vi "module template new.vi"(0 "Static input":T4(array[cluster])=[{"Times"=[947.0, 994.5, 1000.0], "Voltages"=[2.0, -0.5, 2.0], "Enable Ch"=TRUE, "Hinge Points"=3}, {"Times"=[947.0, 994.5, 1000.0], "Voltages"=[-1.0, 0.0, 2.0], "Enable Ch"=TRUE, "Hinge Points"=3}, {"Times"=[947.0, 994.5, 1000.0], "Voltages"=[2.0, -1.0, 2.0], "Enable Ch"=TRUE, "Hinge Points"=3}, {"Times"=[948.5, 1000.0], "Voltages"=[0.05, 0.0], "Enable Ch"=TRUE, "Hinge Points"=2}, {"Times"=[1000.0, 2850.0], "Voltages"=[8.0, -0.5], "Enable Ch"=TRUE, "Hinge Points"=2}, {"Times"=[947.0, 1000.0], "Voltages"=[4.6, 4.3], "Enable Ch"=TRUE, "Hinge Points"=2}, {"Times"=[996.0, 999.0, 1400.0, 1402.0, 1404.0, 1406.0, 1408.0, 1410.0, 1412.0, 1414.0, 1416.0, 1418.0, 1420.0, 1422.0, 1424.0, 1426.0, 1428.0, 1430.0, 1432.0, 1434.0, 1436.0, 1438.0, 1440.0, 1442.0, 1444.0, 1446.0, 1448.0, 1450.0, 1452.0, 1454.0, 1456.0, 1458.0, 1460.0, 1462.0, 1464.0, 1466.0, 1468.0, 1470.0, 1472.0, 1474.0, 1476.0, 1478.0, 1480.0, 1482.0, 1484.0, 1486.0, 1488.0, 1490.0, 1492.0, 1494.0, 1496.0, 1498.0, 1500.0], "Voltages"=[0.0, -1.2, -1.2, -1.256, -1.3119999999999998, -1.3679999999999999, -1.424, -1.48, -1.536, -1.5919999999999999, -1.648, -1.704, -1.7599999999999998, -1.8159999999999998, -1.8719999999999999, -1.928, -1.984, -2.04, -2.096, -2.152, -2.208, -2.264, -2.32, -2.376, -2.4319999999999995, -2.4879999999999995, -2.5439999999999996, -2.5999999999999996, -2.6559999999999997, -2.7119999999999997, -2.768, -2.824, -2.88, -2.936, -2.992, -3.048, -3.104, -3.1599999999999997, -3.216, -3.2719999999999994, -3.3279999999999994, -3.3839999999999995, -3.4399999999999995, -3.4959999999999996, -3.5519999999999996, -3.6079999999999997, -3.6639999999999997, -3.7199999999999998, -3.776, -3.832, -3.888, -3.944, -4.0], "Enable Ch"=TRUE, "Hinge Points"=53}, {"Times"=[], "Voltages"=[], "Enable Ch"=FALSE, "Hinge Points"=0}, {"Times"=[], "Voltages"=[], "Enable Ch"=FALSE, "Hinge Points"=0}, {"Times"=[], "Voltages"=[], "Enable Ch"=FALSE, "Hinge Points"=0}, {"Times"=[], "Voltages"=[], "Enable Ch"=FALSE, "Hinge Points"=0}, {"Times"=[], "Voltages"=[], "Enable Ch"=FALSE, "Hinge Points"=0}, {"Times"=[], "Voltages"=[], "Enable Ch"=FALSE, "Hinge Points"=0}, {"Times"=[], "Voltages"=[], "Enable Ch"=FALSE, "Hinge Points"=0}, {"Times"=[], "Voltages"=[], "Enable Ch"=FALSE, "Hinge Points"=0}, {"Times"=[], "Voltages"=[], "Enable Ch"=FALSE, "Hinge Points"=0}] {"Voltages" format="%.2f"; "Times" format="%.2f"}, 1 "Absolute start time (ms)":dbl=2900.0 format="%.3f", 2 "GPIB Input":T1(array[cluster]) {"Module" items=["TTL high                                                                                 ", "TTL low                          ", "Camera Strobe                   ", "CMOT", "Defaults                           ", "Fluorescence pulse           ", "IP trap                         ", "Kinetics OD image          ", "Kinetics picture", "Kinetics probe pulse", "MOT light only                ", "MOT off                                   ", "MOT on                         ", "Move cart                      ", "OD image                     ", "Optical pumping          ", "Picture                             ", "Probe Pulse", "Quadrupole trap             ", "IP off", "Utility Module 02           ", "Utility Module 03           ", "Molasses          ", "Utility Module 04     ", "Utility Module 05     ", "Utility Module 06     ", "Utility Module 07     ", "Utility Module 08     ", "Utility Module 09     ", "Utility Module 10     ", "Static DAC", "GPIB"]; "Abs Start Time" format="%.3f"}, 3 "Read/Write":bool, 5 "Input":i32[][](array[numeric])=[[-1000, 0, 15, 0], [100, 3, 14, 1], [10000, 3, 14, 0], [947000, 0, 11, 1], [947000, 1, 13, 0], [947000, 2, 9, 1], [947000, 2, 9, 1], [947000, 2, 9, 1], [947000, 2, 9, 1], [947100, 2, 9, 0], [947100, 2, 9, 0], [947100, 2, 9, 0], [947100, 2, 9, 0], [948500, 2, 9, 1], [948600, 2, 9, 0], [990000, 0, 0, 0], [992000, 2, 11, 0], [992000, 2, 12, 1], [994000, 0, 9, 0], [994000, 2, 2, 0], [994500, 2, 9, 1], [994500, 2, 9, 1], [994500, 2, 9, 1], [994600, 2, 9, 0], [994600, 2, 9, 0], [994600, 2, 9, 0], [995500, 1, 0, 0], [996000, 2, 9, 1], [996100, 2, 9, 0], [996500, 0, 5, 0], [996500, 1, 1, 0], [996500, 1, 9, 0], [996500, 2, 3, 1], [997000, 0, 3, 1], [998300, 0, 3, 0], [998450, 0, 11, 0], [998450, 1, 13, 1], [998500, 0, 4, 1], [998850, 0, 14, 1], [999000, 2, 9, 1], [999100, 2, 9, 0], [999450, 0, 14, 0], [999500, 0, 4, 0], [999500, 0, 15, 1], [1000000, 0, 0, 1], [1000000, 0, 1, 1], [1000000, 0, 2, 1], [1000000, 0, 5, 1], [1000000, 1, 1, 1], [1000000, 1, 9, 1], [1000000, 2, 7, 1], [1000000, 2, 9, 1], [1000000, 2, 9, 1], [1000000, 2, 9, 1], [1000000, 2, 9, 1], [1000000, 2, 9, 1], [1000000, 2, 9, 1], [1000100, 2, 9, 0], [1000100, 2, 9, 0], [1000100, 2, 9, 0], [1000100, 2, 9, 0], [1000100, 2, 9, 0], [1000100, 2, 9, 0], [1000500, 2, 3, 0], [1001000, 2, 7, 0], [1005000, 0, 2, 0], [1047000, 2, 11, 0], [1047000, 2, 12, 0], [1400000, 2, 9, 1], [1400100, 2, 9, 0], [1402000, 2, 9, 1], [1402100, 2, 9, 0], [1404000, 2, 9, 1], [1404100, 2, 9, 0], [1406000, 2, 9, 1], [1406100, 2, 9, 0], [1408000, 2, 9, 1], [1408100, 2, 9, 0], [1410000, 2, 9, 1], [1410100, 2, 9, 0], [1412000, 2, 9, 1], [1412100, 2, 9, 0], [1414000, 2, 9, 1], [1414100, 2, 9, 0], [1416000, 2, 9, 1], [1416100, 2, 9, 0], [1418000, 2, 9, 1], [1418100, 2, 9, 0], [1420000, 2, 9, 1], [1420100, 2, 9, 0], [1422000, 2, 9, 1], [1422100, 2, 9, 0], [1424000, 2, 9, 1], [1424100, 2, 9, 0], [1426000, 2, 9, 1], [1426100, 2, 9, 0], [1428000, 2, 9, 1], [1428100, 2, 9, 0], [1430000, 2, 9, 1], [1430100, 2, 9, 0], [1432000, 2, 9, 1], [1432100, 2, 9, 0], [1434000, 2, 9, 1], [1434100, 2, 9, 0], [1436000, 2, 9, 1], [1436100, 2, 9, 0], [1438000, 2, 9, 1], [1438100, 2, 9, 0], [1440000, 2, 9, 1], [1440100, 2, 9, 0], [1442000, 2, 9, 1], [1442100, 2, 9, 0], [1444000, 2, 9, 1], [1444100, 2, 9, 0], [1446000, 2, 9, 1], [1446100, 2, 9, 0], [1448000, 2, 9, 1], [1448100, 2, 9, 0], [1450000, 2, 9, 1], [1450100, 2, 9, 0], [1452000, 2, 9, 1], [1452100, 2, 9, 0], [1454000, 2, 9, 1], [1454100, 2, 9, 0], [1456000, 2, 9, 1], [1456100, 2, 9, 0], [1458000, 2, 9, 1], [1458100, 2, 9, 0], [1460000, 2, 9, 1], [1460100, 2, 9, 0], [1462000, 2, 9, 1], [1462100, 2, 9, 0], [1464000, 2, 9, 1], [1464100, 2, 9, 0], [1466000, 2, 9, 1], [1466100, 2, 9, 0], [1468000, 2, 9, 1], [1468100, 2, 9, 0], [1470000, 2, 9, 1], [1470100, 2, 9, 0], [1472000, 2, 9, 1], [1472100, 2, 9, 0], [1474000, 2, 9, 1], [1474100, 2, 9, 0], [1476000, 2, 9, 1], [1476100, 2, 9, 0], [1478000, 2, 9, 1], [1478100, 2, 9, 0], [1480000, 2, 9, 1], [1480100, 2, 9, 0], [1482000, 2, 9, 1], [1482100, 2, 9, 0], [1484000, 2, 9, 1], [1484100, 2, 9, 0], [1486000, 2, 9, 1], [1486100, 2, 9, 0], [1488000, 2, 9, 1], [1488100, 2, 9, 0], [1490000, 2, 9, 1], [1490100, 2, 9, 0], [1492000, 2, 9, 1], [1492100, 2, 9, 0], [1494000, 2, 9, 1], [1494100, 2, 9, 0], [1496000, 2, 9, 1], [1496100, 2, 9, 0], [1498000, 2, 9, 1], [1498100, 2, 9, 0], [1500000, 2, 9, 1], [1500100, 2, 9, 0], [2400000, 0, 1, 0], [2850000, 2, 9, 1], [2850100, 2, 9, 0]], 7 "Static DAC Linear Ramps":T3(array[cluster])=[{"Write Ramp?"=TRUE, "DAC Channel"=6, "Ramp begin"=400.0, "Ramp end"=500.0, "start value"=-1.2, "end value"=-4.0, "steps"=50}] {"end value" format="%_6g"; "start value" format="%_6g"; "Ramp end" format="%_6g"; "Ramp begin" format="%_6g"; "DAC Channel" items=["0", "1", "2", "3", "4", "5", "6", "7", "8", "9", "10", "11", "12", "13", "14", "0"]}, 9 "Manual Array":T5(array[cluster])=[{"Time2 (ms)"=0.0, "Port2"=1, "Line2"=1, "Comments2"="master switch to coils on", "Value2"=TRUE, "Enable2"=TRUE, "DAC value"=0.0}, {"Time2 (ms)"=-1.0, "Port2"=4, "Line2"=6, "Comments2"="Q trap current to 120A", "Value2"=FALSE, "Enable2"=TRUE, "DAC value"=-1.2}, {"Time2 (ms)"=0.0, "Port2"=4, "Line2"=0, "Comments2"="E/W shim off for Qtrap", "Value2"=FALSE, "Enable2"=TRUE, "DAC value"=2.0}, {"Time2 (ms)"=0.0, "Port2"=4, "Line2"=1, "Comments2"="U/D shim off for Qtrap", "Value2"=FALSE, "Enable2"=TRUE, "DAC value"=2.0}, {"Time2 (ms)"=0.0, "Port2"=4, "Line2"=2, "Comments2"="N/S shim off for Qtrap", "Value2"=FALSE, "Enable2"=TRUE, "DAC value"=2.0}, {"Time2 (ms)"=0.0, "Port2"=0, "Line2"=2, "Comments2"="fast turn on (IGBT on)", "Value2"=TRUE, "Enable2"=TRUE, "DAC value"=0.0}, {"Time2 (ms)"=5.0, "Port2"=0, "Line2"=2, "Comments2"="IGBT off", "Value2"=FALSE, "Enable2"=TRUE, "DAC value"=0.0}] {"Line2" items=["0", "1", "2", "3", "4", "5", "6", "7", "8", "9", "10", "11", "12", "13", "14", "15"]; "Port2" items=["A", "B", "C", "D", "DAC", "GPIB"]; "Time2 (ms)" format="%.3f"}, 10 "Do Write/Read":bool, 12 "Do this?":bool=TRUE, 14 "filename":string="quad trap") -> (4 "Static output":T4(array[cluster])=[{"Times"=[947.0, 994.5, 1000.0, 2900.0], "Voltages"=[2.0, -0.5, 2.0, 2.0], "Enable Ch"=TRUE, "Hinge Points"=4}, {"Times"=[947.0, 994.5, 1000.0, 2900.0], "Voltages"=[-1.0, 0.0, 2.0, 2.0], "Enable Ch"=TRUE, "Hinge Points"=4}, {"Times"=[947.0, 994.5, 1000.0, 2900.0], "Voltages"=[2.0, -1.0, 2.0, 2.0], "Enable Ch"=TRUE, "Hinge Points"=4}, {"Times"=[948.5, 1000.0], "Voltages"=[0.05, 0.0], "Enable Ch"=TRUE, "Hinge Points"=2}, {"Times"=[1000.0, 2850.0], "Voltages"=[8.0, -0.5], "Enable Ch"=TRUE, "Hinge Points"=2}, {"Times"=[947.0, 1000.0], "Voltages"=[4.6, 4.3], "Enable Ch"=TRUE, "Hinge Points"=2}, {"Times"=[996.0, 999.0, 1400.0, 1402.0, 1404.0, 1406.0, 1408.0, 1410.0, 1412.0, 1414.0, 1416.0, 1418.0, 1420.0, 1422.0, 1424.0, 1426.0, 1428.0, 1430.0, 1432.0, 1434.0, 1436.0, 1438.0, 1440.0, 1442.0, 1444.0, 1446.0, 1448.0, 1450.0, 1452.0, 1454.0, 1456.0, 1458.0, 1460.0, 1462.0, 1464.0, 1466.0, 1468.0, 1470.0, 1472.0, 1474.0, 1476.0, 1478.0, 1480.0, 1482.0, 1484.0, 1486.0, 1488.0, 1490.0, 1492.0, 1494.0, 1496.0, 1498.0, 1500.0, 2899.0, 3300.0, 3302.0, 3304.0, 3306.0, 3308.0, 3310.0, 3312.0, 3314.0, 3316.0, 3318.0, 3320.0, 3322.0, 3324.0, 3326.0, 3328.0, 3330.0, 3332.0, 3334.0, 3336.0, 3338.0, 3340.0, 3342.0, 3344.0, 3346.0, 3348.0, 3350.0, 3352.0, 3354.0, 3356.0, 3358.0, 3360.0, 3362.0, 3364.0, 3366.0, 3368.0, 3370.0, 3372.0, 3374.0, 3376.0, 3378.0, 3380.0, 3382.0, 3384.0, 3386.0, 3388.0, 3390.0, 3392.0, 3394.0, 3396.0, 3398.0, 3400.0], "Voltages"=[0.0, -1.2, -1.2, -1.256, -1.3119999999999998, -1.3679999999999999, -1.424, -1.48, -1.536, -1.5919999999999999, -1.648, -1.704, -1.7599999999999998, -1.8159999999999998, -1.8719999999999999, -1.928, -1.984, -2.04, -2.096, -2.152, -2.208, -2.264, -2.32, -2.376, -2.4319999999999995, -2.4879999999999995, -2.5439999999999996, -2.5999999999999996, -2.6559999999999997, -2.7119999999999997, -2.768, -2.824, -2.88, -2.936, -2.992, -3.048, -3.104, -3.1599999999999997, -3.216, -3.2719999999999994, -3.3279999999999994, -3.3839999999999995, -3.4399999999999995, -3.4959999999999996, -3.5519999999999996, -3.6079999999999997, -3.6639999999999997, -3.7199999999999998, -3.776, -3.832, -3.888, -3.944, -4.0, -1.2, -1.2, -1.256, -1.3119999999999998, -1.3679999999999999, -1.424, -1.48, -1.536, -1.5919999999999999, -1.648, -1.704, -1.7599999999999998, -1.8159999999999998, -1.8719999999999999, -1.928, -1.984, -2.04, -2.096, -2.152, -2.208, -2.264, -2.32, -2.376, -2.4319999999999995, -2.4879999999999995, -2.5439999999999996, -2.5999999999999996, -2.6559999999999997, -2.7119999999999997, -2.768, -2.824, -2.88, -2.936, -2.992, -3.048, -3.104, -3.1599999999999997, -3.216, -3.2719999999999994, -3.3279999999999994, -3.3839999999999995, -3.4399999999999995, -3.4959999999999996, -3.5519999999999996, -3.6079999999999997, -3.6639999999999997, -3.7199999999999998, -3.776, -3.832, -3.888, -3.944, -4.0], "Enable Ch"=TRUE, "Hinge Points"=105}, {"Times"=[], "Voltages"=[], "Enable Ch"=FALSE, "Hinge Points"=0}, {"Times"=[], "Voltages"=[], "Enable Ch"=FALSE, "Hinge Points"=0}, {"Times"=[], "Voltages"=[], "Enable Ch"=FALSE, "Hinge Points"=0}, {"Times"=[], "Voltages"=[], "Enable Ch"=FALSE, "Hinge Points"=0}, {"Times"=[], "Voltages"=[], "Enable Ch"=FALSE, "Hinge Points"=0}, {"Times"=[], "Voltages"=[], "Enable Ch"=FALSE, "Hinge Points"=0}, {"Times"=[], "Voltages"=[], "Enable Ch"=FALSE, "Hinge Points"=0}, {"Times"=[], "Voltages"=[], "Enable Ch"=FALSE, "Hinge Points"=0}, {"Times"=[], "Voltages"=[], "Enable Ch"=FALSE, "Hinge Points"=0}] {"Voltages" format="%.2f"; "Times" format="%.2f"}, 6 "Output":i32[][](array[numeric])=[[3400100, 2, 9, 0], [3400000, 2, 9, 1], [3398100, 2, 9, 0], [3398000, 2, 9, 1], [3396100, 2, 9, 0], [3396000, 2, 9, 1], [3394100, 2, 9, 0], [3394000, 2, 9, 1], [3392100, 2, 9, 0], [3392000, 2, 9, 1], [3390100, 2, 9, 0], [3390000, 2, 9, 1], [3388100, 2, 9, 0], [3388000, 2, 9, 1], [3386100, 2, 9, 0], [3386000, 2, 9, 1], [3384100, 2, 9, 0], [3384000, 2, 9, 1], [3382100, 2, 9, 0], [3382000, 2, 9, 1], [3380100, 2, 9, 0], [3380000, 2, 9, 1], [3378100, 2, 9, 0], [3378000, 2, 9, 1], [3376100, 2, 9, 0], [3376000, 2, 9, 1], [3374100, 2, 9, 0], [3374000, 2, 9, 1], [3372100, 2, 9, 0], [3372000, 2, 9, 1], [3370100, 2, 9, 0], [3370000, 2, 9, 1], [3368100, 2, 9, 0], [3368000, 2, 9, 1], [3366100, 2, 9, 0], [3366000, 2, 9, 1], [3364100, 2, 9, 0], [3364000, 2, 9, 1], [3362100, 2, 9, 0], [3362000, 2, 9, 1], [3360100, 2, 9, 0], [3360000, 2, 9, 1], [3358100, 2, 9, 0], [3358000, 2, 9, 1], [3356100, 2, 9, 0], [3356000, 2, 9, 1], [3354100, 2, 9, 0], [3354000, 2, 9, 1], [3352100, 2, 9, 0], [3352000, 2, 9, 1], [3350100, 2, 9, 0], [3350000, 2, 9, 1], [3348100, 2, 9, 0], [3348000, 2, 9, 1], [3346100, 2, 9, 0], [3346000, 2, 9, 1], [3344100, 2, 9, 0], [3344000, 2, 9, 1], [3342100, 2, 9, 0], [3342000, 2, 9, 1], [3340100, 2, 9, 0], [3340000, 2, 9, 1], [3338100, 2, 9, 0], [3338000, 2, 9, 1], [3336100, 2, 9, 0], [3336000, 2, 9, 1], [3334100, 2, 9, 0], [3334000, 2, 9, 1], [3332100, 2, 9, 0], [3332000, 2, 9, 1], [3330100, 2, 9, 0], [3330000, 2, 9, 1], [3328100, 2, 9, 0], [3328000, 2, 9, 1], [3326100, 2, 9, 0], [3326000, 2, 9, 1], [3324100, 2, 9, 0], [3324000, 2, 9, 1], [3322100, 2, 9, 0], [3322000, 2, 9, 1], [3320100, 2, 9, 0], [3320000, 2, 9, 1], [3318100, 2, 9, 0], [3318000, 2, 9, 1], [3316100, 2, 9, 0], [3316000, 2, 9, 1], [3314100, 2, 9, 0], [3314000, 2, 9, 1], [3312100, 2, 9, 0], [3312000, 2, 9, 1], [3310100, 2, 9, 0], [3310000, 2, 9, 1], [3308100, 2, 9, 0], [3308000, 2, 9, 1], [3306100, 2, 9, 0], [3306000, 2, 9, 1], [3304100, 2, 9, 0], [3304000, 2, 9, 1], [3302100, 2, 9, 0], [3302000, 2, 9, 1], [3300100, 2, 9, 0], [3300000, 2, 9, 1], [2900100, 2, 9, 0], [2900000, 2, 9, 1], [2900100, 2, 9, 0], [2900000, 2, 9, 1], [2900100, 2, 9, 0], [2900000, 2, 9, 1], [2899100, 2, 9, 0], [2899000, 2, 9, 1], [-1000, 0, 15, 0], [100, 3, 14, 1], [10000, 3, 14, 0], [947000, 0, 11, 1], [947000, 1, 13, 0], [947000, 2, 9, 1], [947000, 2, 9, 1], [947000, 2, 9, 1], [947000, 2, 9, 1], [947100, 2, 9, 0], [947100, 2, 9, 0], [947100, 2, 9, 0], [947100, 2, 9, 0], [948500, 2, 9, 1], [948600, 2, 9, 0], [990000, 0, 0, 0], [992000, 2, 11, 0], [992000, 2, 12, 1], [994000, 0, 9, 0], [994000, 2, 2, 0], [994500, 2, 9, 1], [994500, 2, 9, 1], [994500, 2, 9, 1], [994600, 2, 9, 0], [994600, 2, 9, 0], [994600, 2, 9, 0], [995500, 1, 0, 0], [996000, 2, 9, 1], [996100, 2, 9, 0], [996500, 0, 5, 0], [996500, 1, 1, 0], [996500, 1, 9, 0], [996500, 2, 3, 1], [997000, 0, 3, 1], [998300, 0, 3, 0], [998450, 0, 11, 0], [998450, 1, 13, 1], [998500, 0, 4, 1], [998850, 0, 14, 1], [999000, 2, 9, 1], [999100, 2, 9, 0], [999450, 0, 14, 0], [999500, 0, 4, 0], [999500, 0, 15, 1], [1000000, 0, 0, 1], [1000000, 0, 1, 1], [1000000, 0, 2, 1], [1000000, 0, 5, 1], [1000000, 1, 1, 1], [1000000, 1, 9, 1], [1000000, 2, 7, 1], [1000000, 2, 9, 1], [1000000, 2, 9, 1], [1000000, 2, 9, 1], [1000000, 2, 9, 1], [1000000, 2, 9, 1], [1000000, 2, 9, 1], [1000100, 2, 9, 0], [1000100, 2, 9, 0], [1000100, 2, 9, 0], [1000100, 2, 9, 0], [1000100, 2, 9, 0], [1000100, 2, 9, 0], [1000500, 2, 3, 0], [1001000, 2, 7, 0], [1005000, 0, 2, 0], [1047000, 2, 11, 0], [1047000, 2, 12, 0], [1400000, 2, 9, 1], [1400100, 2, 9, 0], [1402000, 2, 9, 1], [1402100, 2, 9, 0], [1404000, 2, 9, 1], [1404100, 2, 9, 0], [1406000, 2, 9, 1], [1406100, 2, 9, 0], [1408000, 2, 9, 1], [1408100, 2, 9, 0], [1410000, 2, 9, 1], [1410100, 2, 9, 0], [1412000, 2, 9, 1], [1412100, 2, 9, 0], [1414000, 2, 9, 1], [1414100, 2, 9, 0], [1416000, 2, 9, 1], [1416100, 2, 9, 0], [1418000, 2, 9, 1], [1418100, 2, 9, 0], [1420000, 2, 9, 1], [1420100, 2, 9, 0], [1422000, 2, 9, 1], [1422100, 2, 9, 0], [1424000, 2, 9, 1], [1424100, 2, 9, 0], [1426000, 2, 9, 1], [1426100, 2, 9, 0], [1428000, 2, 9, 1], [1428100, 2, 9, 0], [1430000, 2, 9, 1], [1430100, 2, 9, 0], [1432000, 2, 9, 1], [1432100, 2, 9, 0], [1434000, 2, 9, 1], [1434100, 2, 9, 0], [1436000, 2, 9, 1], [1436100, 2, 9, 0], [1438000, 2, 9, 1], [1438100, 2, 9, 0], [1440000, 2, 9, 1], [1440100, 2, 9, 0], [1442000, 2, 9, 1], [1442100, 2, 9, 0], [1444000, 2, 9, 1], [1444100, 2, 9, 0], [1446000, 2, 9, 1], [1446100, 2, 9, 0], [1448000, 2, 9, 1], [1448100, 2, 9, 0], [1450000, 2, 9, 1], [1450100, 2, 9, 0], [1452000, 2, 9, 1], [1452100, 2, 9, 0], [1454000, 2, 9, 1], [1454100, 2, 9, 0], [1456000, 2, 9, 1], [1456100, 2, 9, 0], [1458000, 2, 9, 1], [1458100, 2, 9, 0], [1460000, 2, 9, 1], [1460100, 2, 9, 0], [1462000, 2, 9, 1], [1462100, 2, 9, 0], [1464000, 2, 9, 1], [1464100, 2, 9, 0], [1466000, 2, 9, 1], [1466100, 2, 9, 0], [1468000, 2, 9, 1], [1468100, 2, 9, 0], [1470000, 2, 9, 1], [1470100, 2, 9, 0], [1472000, 2, 9, 1], [1472100, 2, 9, 0], [1474000, 2, 9, 1], [1474100, 2, 9, 0], [1476000, 2, 9, 1], [1476100, 2, 9, 0], [1478000, 2, 9, 1], [1478100, 2, 9, 0], [1480000, 2, 9, 1], [1480100, 2, 9, 0], [1482000, 2, 9, 1], [1482100, 2, 9, 0], [1484000, 2, 9, 1], [1484100, 2, 9, 0], [1486000, 2, 9, 1], [1486100, 2, 9, 0], [1488000, 2, 9, 1], [1488100, 2, 9, 0], [1490000, 2, 9, 1], [1490100, 2, 9, 0], [1492000, 2, 9, 1], [1492100, 2, 9, 0], [1494000, 2, 9, 1], [1494100, 2, 9, 0], [1496000, 2, 9, 1], [1496100, 2, 9, 0], [1498000, 2, 9, 1], [1498100, 2, 9, 0], [1500000, 2, 9, 1], [1500100, 2, 9, 0], [2400000, 0, 1, 0], [2850000, 2, 9, 1], [2850100, 2, 9, 0], [2900000, 0, 2, 1], [2900000, 1, 1, 1], [2905000, 0, 2, 0]], 13 "GPIB Output":T1(array[cluster]) {"Module" items=["TTL high                                                                                 ", "TTL low                          ", "Camera Strobe                   ", "CMOT", "Defaults                           ", "Fluorescence pulse           ", "IP trap                         ", "Kinetics OD image          ", "Kinetics picture", "Kinetics probe pulse", "MOT light only                ", "MOT off                                   ", "MOT on                         ", "Move cart                      ", "OD image                     ", "Optical pumping          ", "Picture                             ", "Probe Pulse", "Quadrupole trap             ", "IP off", "Utility Module 02           ", "Utility Module 03           ", "Molasses          ", "Utility Module 04     ", "Utility Module 05     ", "Utility Module 06     ", "Utility Module 07     ", "Utility Module 08     ", "Utility Module 09     ", "Utility Module 10     ", "Static DAC", "GPIB"]; "Abs Start Time" format="%.3f"}, 15 "Saved Cluster":T2={"Manual Array"=[{"Time2 (ms)"=0.0, "Port2"=1, "Line2"=1, "Comments2"="master switch to coils on", "Value2"=TRUE, "Enable2"=TRUE, "DAC value"=0.0}, {"Time2 (ms)"=-1.0, "Port2"=4, "Line2"=6, "Comments2"="Q trap current to 120A", "Value2"=FALSE, "Enable2"=TRUE, "DAC value"=-1.2}, {"Time2 (ms)"=0.0, "Port2"=4, "Line2"=0, "Comments2"="E/W shim off for Qtrap", "Value2"=FALSE, "Enable2"=TRUE, "DAC value"=2.0}, {"Time2 (ms)"=0.0, "Port2"=4, "Line2"=1, "Comments2"="U/D shim off for Qtrap", "Value2"=FALSE, "Enable2"=TRUE, "DAC value"=2.0}, {"Time2 (ms)"=0.0, "Port2"=4, "Line2"=2, "Comments2"="N/S shim off for Qtrap", "Value2"=FALSE, "Enable2"=TRUE, "DAC value"=2.0}, {"Time2 (ms)"=0.0, "Port2"=0, "Line2"=2, "Comments2"="fast turn on (IGBT on)", "Value2"=TRUE, "Enable2"=TRUE, "DAC value"=0.0}, {"Time2 (ms)"=5.0, "Port2"=0, "Line2"=2, "Comments2"="IGBT off", "Value2"=FALSE, "Enable2"=TRUE, "DAC value"=0.0}], "Static DAC Linear Ramps"=[{"Write Ramp?"=TRUE, "DAC Channel"=6, "Ramp begin"=400.0, "Ramp end"=500.0, "start value"=-1.2, "end value"=-4.0, "steps"=50}]})   [LabVIEW 2015]
uses:
  globals and logs/modules globals.vi
  globals and logs/board parameters.vi
  globals and logs/static dac defaults.vi
panel:
  in  "Load modules from backup":bool
  out "Path":path=path "E:/Debbie/experiment stuff/B231/24 Experiment Control/modules and sub-vi's/quad trap"
  out "appended path":path=path "E:/Debbie/experiment stuff/B231/24 Experiment Control/modules and sub-vi's/backups/Helmholtz1 28_Apr_2006"
  out "Comments":string[](array[string])=["master switch to coils on", "fast turn on (IGBT on)", "IGBT off"]
  out "Value":bool[](array[boolean])=[TRUE, TRUE, FALSE]
  out "Line":i32[](array[numeric])=[1, 2, 2]
  out "Port":i32[](array[numeric])=[1, 0, 0]
  out "Time":dbl[](array[numeric])=[0.0, 0.0, 5.0] format="%.3f"
  # "manual button (not connected on icon)\nIf you set this to True, be sure to set it back to False afterward."
  # "Time                   Port        Line       Value  Enable  DAC voltage  Comments"
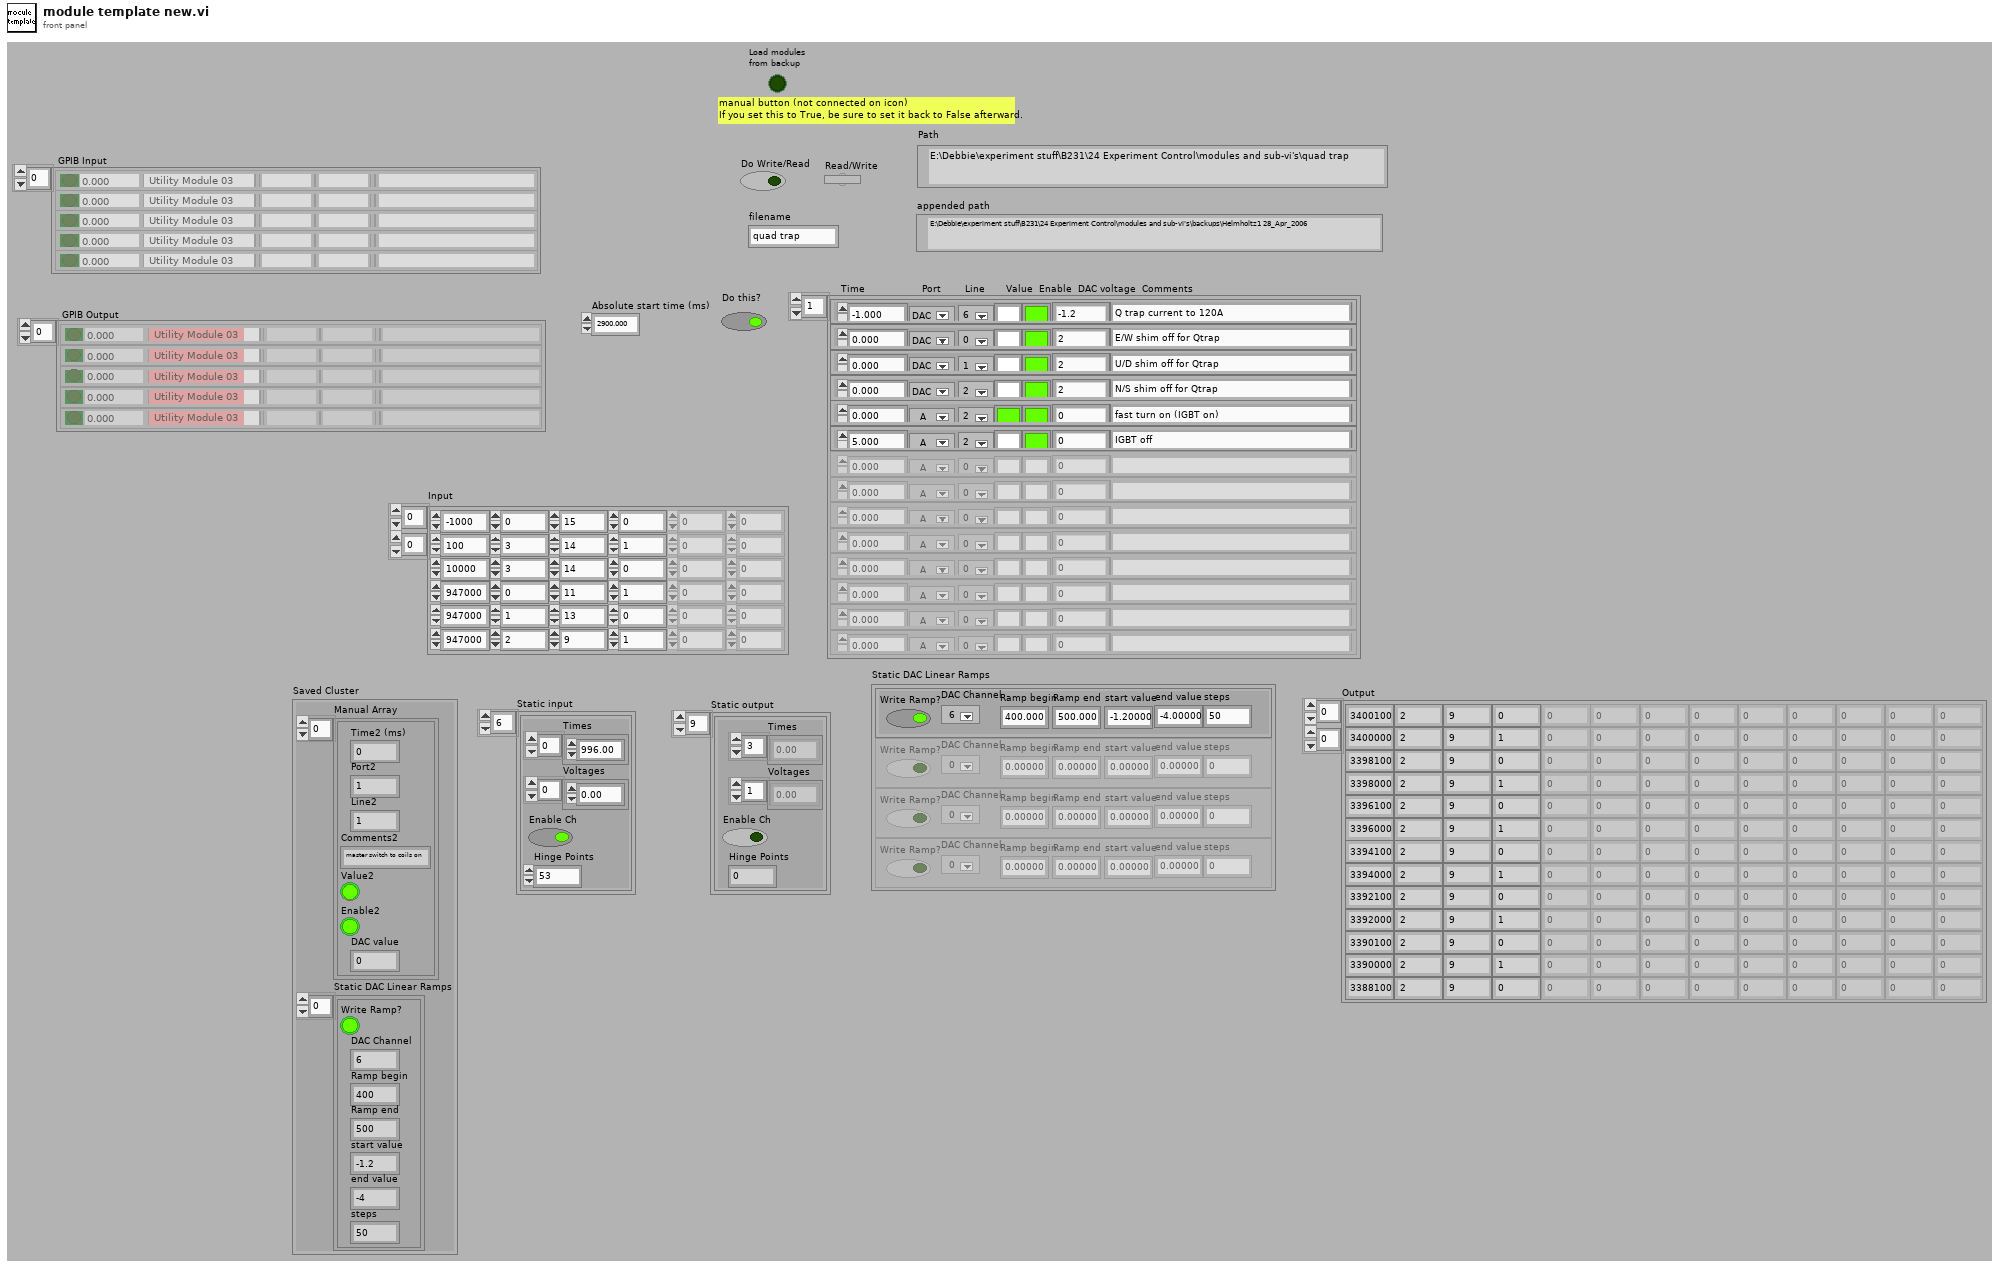
[diagram p1: front panel]
types:
  T1 = cluster{"Enable":bool, "Abs Start Time":dbl, "Module":u16, "String":string, "Array":string[]}[]
  T2 = cluster{"Manual Array":cluster{"Time2 (ms)":dbl, "Port2":u16, "Line2":u16, "Comments2":string, "Value2":bool, "Enable2":bool, "DAC value":dbl}[], "Static DAC Linear Ramps":cluster{"Write Ramp?":bool, "DAC Channel":i16, "Ramp begin":dbl, "Ramp end":dbl, "start value":dbl, "end value":dbl, "steps":i16}[]}
  T3 = cluster{"Write Ramp?":bool, "DAC Channel":i16, "Ramp begin":dbl, "Ramp end":dbl, "start value":dbl, "end value":dbl, "steps":i16}[]
  T4 = cluster{"Times":dbl[], "Voltages":dbl[], "Enable Ch":bool, "Hinge Points":u8}[]
  T5 = cluster{"Time2 (ms)":dbl, "Port2":u16, "Line2":u16, "Comments2":string, "Value2":bool, "Enable2":bool, "DAC value":dbl}[]
  T6 = enum32{"existing file", "new file", "new or existing file", "existing dir", "new dir", "new or existing dir", "existing file (use LLBs)", "new file (use LLBs)", "new or existing file (use LLBs)", "new or existing file or directory (use LLBs)"}
  T7 = enum16{"open", "replace", "create", "open or create", "replace or create", "replace or create with confirmation"}
  T8 = cluster{"Time2 (ms)":dbl, "Port2":u16, "Line2":u16, "Comments2":string, "Value2":bool, "Enable2":bool, "DAC value":dbl}
  T9 = cluster{"Enable":bool, "Abs Start Time":dbl, "Module":u16, "String":string, "Array":string[]}
  T10 = cluster{"Times":dbl[], "Voltages":dbl[], "Enable Ch":bool, "Hinge Points":u8}
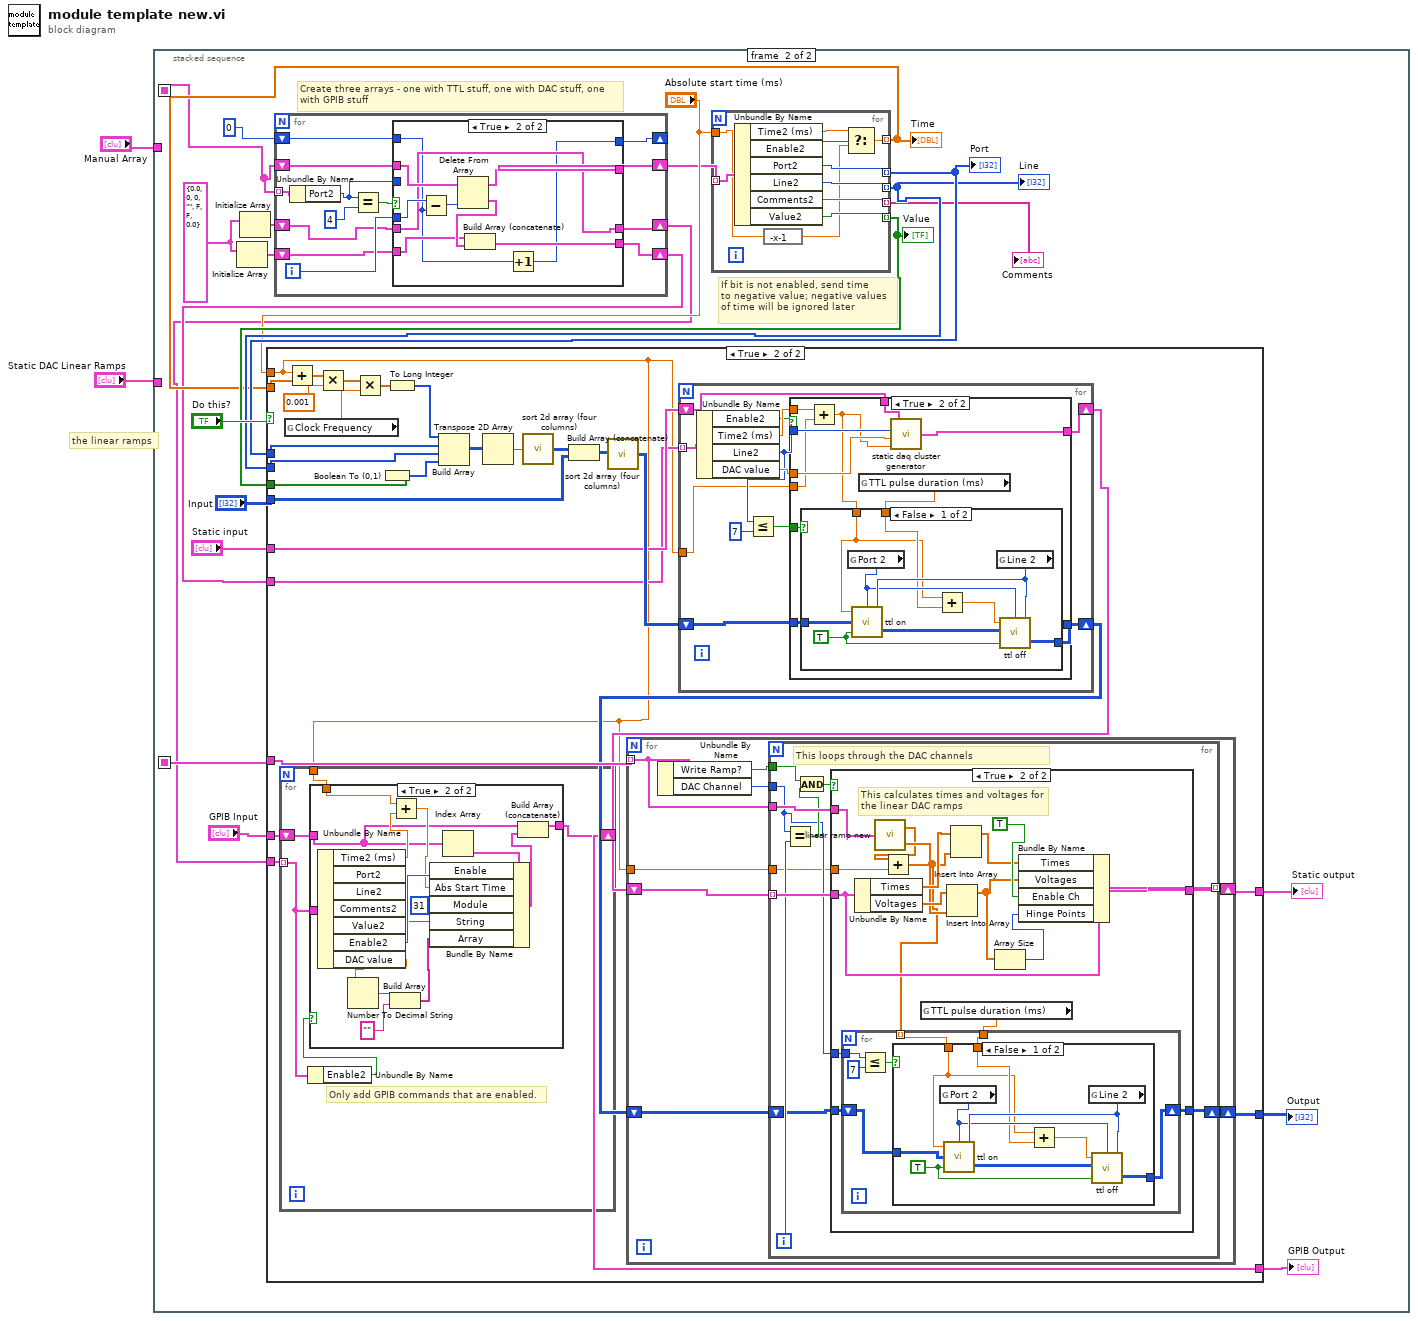
[diagram p0: block diagram]
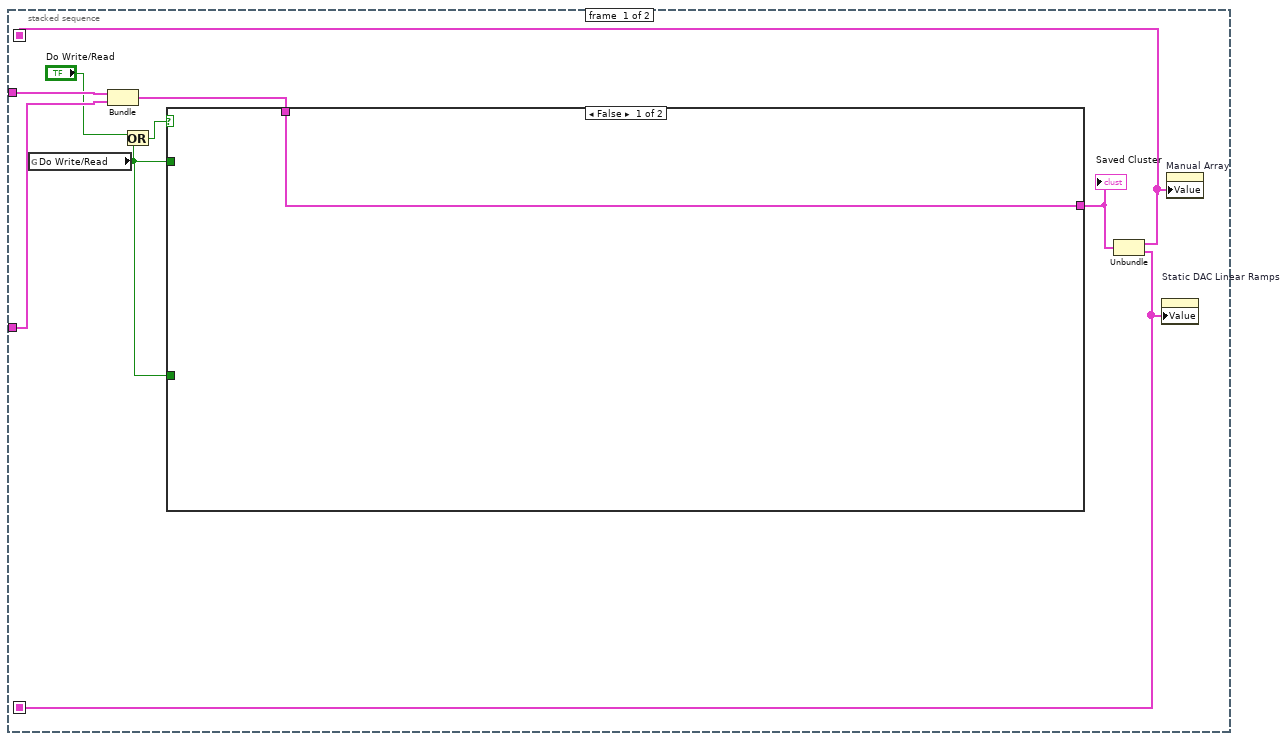
[diagram p2: hidden frame]
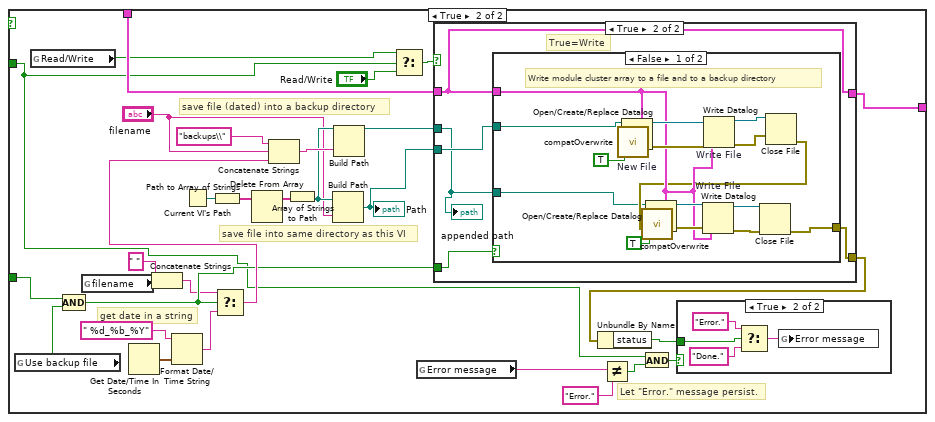
[diagram p3: hidden frame]
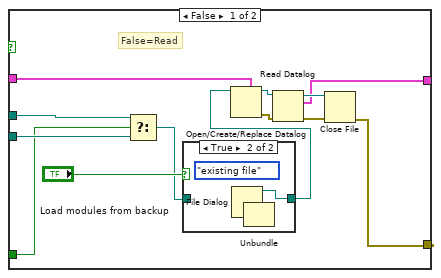
[diagram p5: hidden frame]
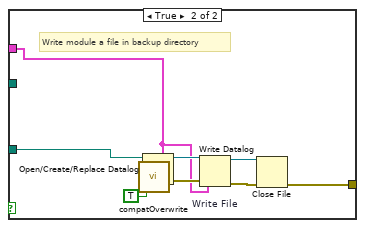
[diagram p7: hidden frame]
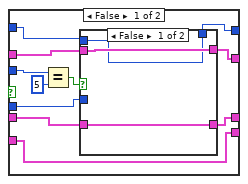
[diagram p8: hidden frame]
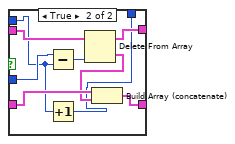
[diagram p9: hidden frame]
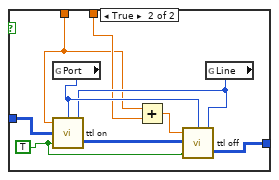
[diagram p13: hidden frame]
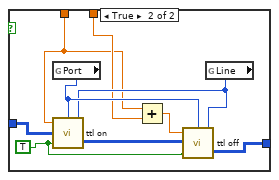
[diagram p15: hidden frame]
diagram:
  # "the linear ramps"
  n1 = stacked-sequence {
    seq-local: [w6 _] -> [_ w104]
    seq-local: [w7 _] -> [_ w106]
    tunnel: "Manual Array" -> [w10 _]
    tunnel: "Static DAC Linear Ramps" -> [w9 _]
    frame #0 {
      n2 = global read "modules globals.vi" "Do Write/Read"() -> (w3:bool)
      n3 = Bundle("Manual Array"=w10, "Static DAC Linear Ramps"=w9) -> (w11:T2)  [unwired: 1 in]
      n4 = Or(x="Do Write/Read", y=w3) -> (x .or. y?=w5:bool)
      n5 = case shown="False" w5 {
        tunnel: w11 -> [w12 w34]
        tunnel: [w12 w33] -> w8
        tunnel: w3 -> [_ w14]
        tunnel: w3 -> [_ w13]
        frame False {
        }
        frame True {
          # "Let \"Error.\" message persist."
          # "get date in a string"
          # "save file (dated) into a backup directory"
          # "save file into same directory as this VI"
          n6 = global read "modules globals.vi" "Use backup file"() -> (w30:bool)
          n7 = global read "modules globals.vi" "Read/Write"() -> (w29:bool)
          n8 = Compound Arithmetic op=AND(w13, w30) -> (w24:bool)
          n9 = global read "modules globals.vi" "filename"() -> (w20:string)
          n10 = Get Date/Time In Seconds() -> (seconds since 1Jan1904=w27:timestamp)
          n11 = Concatenate Strings(" " ("string"), w20) -> (w19:string)
          n12 = Format Date/Time String(time format string (%c)=" %d_%b_%Y", seconds (now)=w27) -> (date/time string=w26:string)  [unwired: 1 in]
          n13 = Current VI's Path() -> (path=w35:path)
          n14 = Path to Array of Strings(0:w35) -> (2:w36:string[])  [unwired: 1 out]
          n15 = Select(t=w19, s=w24, f=w26) -> (s? t:f=w25:string)
          n16 = Delete From Array(array=w36) -> (array with subset deleted=w37:string[])  [unwired: 2 in, 1 out]
          n17 = Concatenate Strings("backups\\" ("Substring"), "filename", w25) -> (w41:string)
          n18 = Array of Strings to Path(0:w37) -> (2:w40:path)  [unwired: 1 in]
          n19 = Build Path(base path=w40, name or relative path="filename") -> (appended path=w42:path)
          "Path" <- w42
          n20 = Build Path(base path=w40, name or relative path=w41) -> (appended path=w43:path)
          n21 = Select(t=w29, s=w14, f="Read/Write") -> (s? t:f=w31:bool)
          n22 = global read "modules globals.vi" "Error message"() -> (w18:string)
          n23 = case shown="True" w31 {
            tunnel: [w60 w68] -> w23
            tunnel: w42 -> [w53 w67]
            tunnel: w43 -> [w51 w65]
            tunnel: w34 -> [w56 w66]
            tunnel: [w54 w66] -> w33
            tunnel: w24 -> [w52 w64]
            frame False {
              # "False=Read"
              n24 = Select(t=w51, s=w52, f=w53) -> (s? t:f=w49:path)
              n25 = case shown="True" "Load modules from backup" {
                tunnel: w49 -> [w61 _]
                tunnel: [w61 w63] -> w48
                frame False {
                }
                frame True {
                  (unwired) T6."existing file" ("select mode (2)")
                  n26 = File Dialog() -> (0:w62:errorcluster, 3:w63:path)  [unwired: 7 in, 2 out]
                  n27 = Unbundle(w62) -> ()  [unwired: 3 out]
                }
              }
              n28 = Open/Create/Replace Datalog(5:w56, 11:w48) -> (0:w58:errorcluster, 3:w55:refnum<k1>)  [unwired: 4 in, 1 out]
              n29 = Read Datalog(4:w58, 7:w55) -> (0:w59:errorcluster, 2:w54:T2, 3:w57:refnum<k1>)  [unwired: 1 in]
              n30 = Close File(refnum=w57, error in=w59) -> (error out=w60:errorcluster)  [unwired: 1 out]
            }
            frame True {
              # "True=Write"
              n31 = case shown="False" w64 {
                tunnel: [w78 w89] -> w68
                tunnel: w67 -> [w76 _]
                tunnel: w66 -> [w74 w87]
                tunnel: w65 -> [w71 w88]
                frame False {
                  # "Write module cluster array to a file and to a backup directory"
                  n32 = call <vilib>:"compatOverwrite.vi"("overwrite (F)"=TRUE) -> ("overwrite?"=w69:T7)
                  n33 = Open/Create/Replace Datalog "New File"(5:w74, 10:w69, 11:w76) -> (0:w81:errorcluster, 3:w75:refnum<k1>)  [unwired: 3 in, 1 out]
                  n34 = call <vilib>:"compatOverwrite.vi"("overwrite (F)"=TRUE) -> ("overwrite?"=w70:T7)
                  n35 = Write Datalog "Write File"(4:w81, 6:w74, 7:w75) -> (0:w82:errorcluster, 3:w84:refnum<k1>)
                  n36 = Close File(refnum=w84, error in=w82) -> (error out=w73:errorcluster)  [unwired: 1 out]
                  n37 = Open/Create/Replace Datalog ("New File")(5:w74, 8:w73, 10:w70, 11:w71) -> (0:w79:errorcluster, 3:w77:refnum<k1>)  [unwired: 2 in, 1 out]
                  n38 = Write Datalog "Write File"(4:w79, 6:w74, 7:w77) -> (0:w80:errorcluster, 3:w83:refnum<k1>)
                  n39 = Close File(refnum=w83, error in=w80) -> (error out=w78:errorcluster)  [unwired: 1 out]
                }
                frame True {
                  # "Write module a file in backup directory"
                  n40 = call <vilib>:"compatOverwrite.vi"("overwrite (F)"=TRUE) -> ("overwrite?"=w86:T7)
                  n41 = Open/Create/Replace Datalog ("New File")(5:w87, 10:w86, 11:w88) -> (0:w92:errorcluster, 3:w91:refnum<k1>)  [unwired: 3 in, 1 out]
                  n42 = Write Datalog "Write File"(4:w92, 6:w87, 7:w91) -> (0:w93:errorcluster, 3:w94:refnum<k1>)
                  n43 = Close File(refnum=w94, error in=w93) -> (error out=w89:errorcluster)  [unwired: 1 out]
                }
              }
              "appended path" <- w65
            }
          }
          n44 = Unbundle By Name(w23) -> ("status"=w22:bool)
          n45 = Not Equal?(x=w18, y="Error." ("Error message")) -> (x != y?=w15:bool)
          n46 = And(x=w14, y=w15) -> (x .and. y?=w16:bool)
          n47 = case shown="True" w16 {
            tunnel: w22 -> [_ w46]
            frame False {
            }
            frame True {
              n48 = Select(t="Error." ("Error message"), s=w46, f="Done." ("Error message")) -> (s? t:f=w47:string)
              n49 = global write "modules globals.vi" "Error message"(w47) -> ()
            }
          }
        }
      }
      "Saved Cluster" <- w8
      n50 = Unbundle(w8) -> ("Manual Array"=w7:T5, "Static DAC Linear Ramps"=w6:T3)
      n51 = property on="Static DAC Linear Ramps" class="Arr (strict)"("Value"=w6) -> ()  [unwired: 2 in, 2 out]
      n52 = property on="Manual Array" class="Arr (strict)"("Value"=w7) -> ()  [unwired: 2 in, 2 out]
    }
    frame #1 {
      w99 = T8 {"Time2 (ms)"=0.0, "Port2"=0, "Line2"=0, "Comments2"="", "Value2"=FALSE, "Enable2"=FALSE, "DAC value"=0.0} ("manual cluster")
      # "Create three arrays - one with TTL stuff, one with DAC stuff, one with GPIB stuff"
      # "If bit is not enabled, send time\nto negative value; negative values\nof time will be ignored later"
      n53 = Initialize Array(w99) -> (w108:T5)  [unwired: 1 in]
      n54 = Initialize Array(w99) -> (w98:T5)  [unwired: 1 in]
      n55 = for {
        tunnel: w106 -> [w123] mode=indexing
        shift-right: [w128] -> w107
        shift-left: w106 -> [w129]
        shift-right: [w121] -> w105
        shift-left: w108 -> [w124]
        shift-right: [w119] -> w97
        shift-left: w98 -> [w120]
        shift-right: [w117] -> _
        shift-left: u16 0 ("y") -> [w118]
        i -> [w125]
        n56 = Unbundle By Name(w123) -> ("Port2"=w122:u16)
        n57 = Equal?(x=w122, y=u16 4) -> (x = y?=w127:bool)
        n58 = case shown="True" w127 {
          tunnel: w129 -> [w138 w162]
          tunnel: [w137 w161] -> w128
          tunnel: w125 -> [w135 w158]
          tunnel: [w133 w159] -> w121
          tunnel: w124 -> [w133 w155]
          tunnel: w122 -> [w139 _]
          tunnel: w120 -> [w134 w156]
          tunnel: [w132 w156] -> w119
          tunnel: w118 -> [w131 w154]
          tunnel: [w130 w153] -> w117
          frame False {
            n59 = Equal?(x=w139, y=u16 5) -> (x = y?=w136:bool)
            n60 = case shown="False" w136 {
              tunnel: w138 -> [w143 w151]
              tunnel: w134 -> [w142 w148]
              tunnel: [w143 w150] -> w137
              tunnel: [w142 w149] -> w132
              tunnel: w135 -> [_ w152]
              tunnel: w131 -> [w141 w145]
              tunnel: [w141 w144] -> w130
              frame False {
              }
              frame True {
                n61 = Subtract(x=w152, y=w145) -> (x-y=w146:i32)
                n62 = Increment(x=w145) -> (x+1=w144:u16)
                n63 = Delete From Array(array=w151, index=w146) -> (deleted portion=w147:T8, array with subset deleted=w150:T5)  [unwired: 1 in]
                n64 = Build Array (concatenate)(w148, w147) -> (w149:T5)
              }
            }
          }
          frame True {
            n65 = Subtract(x=w158, y=w154) -> (x-y=w157:i32)
            n66 = Delete From Array(array=w162, index=w157) -> (deleted portion=w160:T8, array with subset deleted=w161:T5)  [unwired: 1 in]
            n67 = Build Array (concatenate)(w155, w160) -> (w159:T5)
            n68 = Increment(x=w154) -> (x+1=w153:u16)
          }
        }
      }
      n69 = for {
        tunnel: w107 -> [w172] mode=indexing
        tunnel: [w167] -> w111 mode=indexing
        tunnel: [w171] -> w115 mode=indexing
        tunnel: [w170] -> w114 mode=indexing
        tunnel: [w169] -> w113 mode=indexing
        tunnel: [w168] -> w112 mode=indexing
        tunnel: "Absolute start time (ms)" -> [w163]
        n70 = Unbundle By Name(w172) -> ("Time2 (ms)"=w166:dbl, "Enable2"=w164:bool, "Port2"=w171:u16, "Line2"=w170:u16, "Comments2"=w169:string, "Value2"=w168:bool)
        n71 = expression code="-x-1"(w163) -> (w165:dbl)
        n72 = Select(t=w166, s=w164, f=w165) -> (s? t:f=w167:dbl)
      }
      "Time" <- w111
      "Port" <- w115
      "Line" <- w114
      "Comments" <- w113
      "Value" <- w112
      n73 = case shown="True" "Do this?" {
        tunnel: w111 -> [_ w200]
        tunnel: w115 -> [_ w193]
        tunnel: w114 -> [_ w192]
        tunnel: w112 -> [_ w199]
        tunnel: "Static input" -> [w175 w187]
        tunnel: w105 -> [_ w186]
        tunnel: "Absolute start time (ms)" -> [_ w176]
        tunnel: w104 -> [_ w185]
        tunnel: [w175 w183] -> w103
        tunnel: [w174 w180] -> w101
        tunnel: "Input" -> [w174 w182]
        tunnel: "GPIB Input" -> [w173 w178]
        tunnel: w97 -> [_ w179]
        tunnel: [w173 w177] -> w96
        frame False {
        }
        frame True {
          n74 = for {
            tunnel: w179 -> [w205] mode=indexing
            shift-right: [w207] -> w177
            shift-left: w178 -> [w208]
            tunnel: w176 -> [w206]
            # "Only add GPIB commands that are enabled."
            n75 = Unbundle By Name(w205) -> ("Enable2"=w204:bool)
            n76 = case shown="True" w204 {
              tunnel: w208 -> [w209 w210]
              tunnel: [w209 w215] -> w207
              tunnel: w206 -> [_ w214]
              tunnel: w205 -> [_ w211]
              frame False {
              }
              frame True {
                n77 = Unbundle By Name(w211) -> ("Time2 (ms)"=w212:dbl, "Comments2"=w221:string, "Enable2"=w223:bool, "DAC value"=w217:dbl)  [unwired: 3 out]
                n78 = Number To Decimal String(number=w217) -> (decimal integer string=w220:string)  [unwired: 1 in]
                n79 = Build Array(w220, "" ("element")) -> (w218:string[])
                n80 = Add(x=w214, y=w212) -> (x+y=w213:dbl)
                n81 = Index Array(array=w210) -> (element=w224:T9)  [unwired: 1 in]
                n82 = Bundle By Name(cluster=w224, "Enable"=w223, "Abs Start Time"=w213, "Module"=u16 31, "String"=w221, "Array"=w218) -> (w216:T9)
                n83 = Build Array (concatenate)(w210, w216) -> (w215:T1)
              }
            }
          }
          n84 = global read "board parameters.vi" "Clock Frequency"() -> (w201:dbl)
          n85 = Add(x=w176, y=w200) -> (x+y=w197:dbl[])
          n86 = Multiply(x=w197, y=0.001) -> (x*y=w202:dbl[])
          n87 = Multiply(x=w202, y=w201) -> (x*y=w198:dbl[])
          n88 = Boolean To (0,1)(Boolean=w199) -> (0, 1=w191:i16[])
          n89 = To Long Integer(number=w198) -> (32bit integer=w194:i32[])
          n90 = Build Array(w194, w193, w192, w191) -> (w196:i32[][])
          n91 = Transpose 2D Array(2D array=w196) -> (transposed array=w195:i32[][])
          n92 = call "sort 2d array (four columns).vi"("2D array to sort"=w195) -> ("Sorted array"=w190:i32[][])
          n93 = Build Array (concatenate)(w190, w182) -> (w189:i32[][])
          n94 = call "sort 2d array (four columns).vi"("2D array to sort"=w189) -> ("Sorted array"=w188:i32[][])
          n95 = for {
            shift-right: [w293] -> w184
            shift-left: w187 -> [w296]
            tunnel: w186 -> [w297] mode=indexing
            shift-right: [w292] -> w181
            shift-left: w188 -> [w298]
            tunnel: w176 -> [w291]
            n96 = Unbundle By Name(w297) -> ("Enable2"=w289:bool, "Time2 (ms)"=w290:dbl, "Line2"=w294:u16, "DAC value"=w295:dbl)
            n97 = Less Or Equal?(x=w294, y=7) -> (x <= y?=w288:bool)
            n98 = case shown="True" w289 {
              tunnel: w288 -> [_ w312]
              tunnel: w298 -> [w300 w311]
              tunnel: w296 -> [w301 w310]
              tunnel: w295 -> [_ w309]
              tunnel: w294 -> [_ w308]
              tunnel: [w301 w307] -> w293
              tunnel: [w300 w306] -> w292
              tunnel: w291 -> [_ w304]
              tunnel: w290 -> [_ w303]
              frame False {
              }
              frame True {
                n99 = Add(x=w303, y=w304) -> (x+y=w302:dbl)
                n100 = global read "static dac defaults.vi" "TTL pulse duration (ms)"() -> (w305:dbl)
                n101 = case shown="False" w312 {
                  tunnel: w311 -> [w316 w330]
                  tunnel: [w317 w323] -> w306
                  tunnel: w305 -> [w314 w324]
                  tunnel: w302 -> [w313 w322]
                  frame False {
                    w315 = TRUE ("Do this?")
                    n102 = global read "static dac defaults.vi" "Port 2"() -> (w320:i32)
                    n103 = Add(x=w313, y=w314) -> (x+y=w318:dbl)
                    n104 = global read "static dac defaults.vi" "Line 2"() -> (w321:i32)
                    n105 = call "ttl on.vi"("Line"=w321, "Port"=w320, "Do this?"=w315, "Input"=w316, "Absolute start time (ms)"=w313) -> ("Output"=w319:i32[][])
                    n106 = call "ttl off.vi"("Line"=w321, "Port"=w320, "Do this?"=w315, "Input"=w319, "Absolute start time (ms)"=w318) -> ("Output"=w317:i32[][])
                  }
                  frame True {
                    w325 = TRUE ("Do this?")
                    n107 = global read "static dac defaults.vi" "Port"() -> (w327:i32)
                    n108 = Add(x=w322, y=w324) -> (x+y=w329:dbl)
                    n109 = global read "static dac defaults.vi" "Line"() -> (w326:i32)
                    n110 = call "ttl on.vi"("Line"=w326, "Port"=w327, "Do this?"=w325, "Input"=w330, "Absolute start time (ms)"=w322) -> ("Output"=w328:i32[][])
                    n111 = call "ttl off.vi"("Line"=w326, "Port"=w327, "Do this?"=w325, "Input"=w328, "Absolute start time (ms)"=w329) -> ("Output"=w323:i32[][])
                  }
                }
                n112 = call "static daq cluster generator.vi"("time entry"=w302, "voltage entry"=w309, "DAQ channel\n number"=w308, "Input Array"=w310) -> ("Output Array"=w307:T4)
              }
            }
          }
          n113 = for {
            tunnel: w185 -> [w231] mode=indexing
            shift-right: [w229] -> w183
            shift-left: w184 -> [w230]
            shift-right: [w226] -> w180
            shift-left: w181 -> [w227]
            tunnel: w176 -> [w225]
            n114 = Unbundle By Name(w231) -> ("Write Ramp?"=w232:bool, "DAC Channel"=w228:i16)
            n115 = for {
              tunnel: w232 -> [w238]
              tunnel: w231 -> [w243]
              tunnel: w230 -> [w242] mode=indexing
              tunnel: [w241] -> w229 mode=indexing
              tunnel: w228 -> [w237]
              shift-right: [w234] -> w226
              shift-left: w227 -> [w235]
              tunnel: w225 -> [w233]
              i -> [w240]
              # "This loops through the DAC channels"
              n116 = Equal?(x=w237, y=w240) -> (x = y?=w239:bool)
              n117 = And(x=w238, y=w239) -> (x .and. y?=w236:bool)
              n118 = case shown="True" w236 {
                tunnel: w243 -> [_ w262]
                tunnel: w242 -> [w245 w261]
                tunnel: [w245 w255] -> w241
                tunnel: w235 -> [w244 w251]
                tunnel: [w244 w250] -> w234
                tunnel: w237 -> [_ w249]
                tunnel: w233 -> [_ w247]
                frame False {
                }
                frame True {
                  # "This calculates times and voltages for the linear DAC ramps"
                  n119 = Unbundle By Name(w261) -> ("Times"=w260:dbl[], "Voltages"=w259:dbl[])
                  n120 = call "linear ramp new.vi"("Input"=w262) -> ("Time Array"=w248:dbl[], "Volt Array"=w258:dbl[])
                  n121 = Add(x=w248, y=w247) -> (x+y=w246:dbl[])
                  n122 = global read "static dac defaults.vi" "TTL pulse duration (ms)"() -> (w252:dbl)
                  n123 = for {
                    tunnel: w252 -> [w268]
                    tunnel: w246 -> [w267] mode=indexing
                    shift-right: [w265] -> w250
                    shift-left: w251 -> [w266]
                    tunnel: w249 -> [w264]
                    n124 = Less Or Equal?(x=w264, y=7) -> (x <= y?=w263:bool)
                    n125 = case shown="False" w263 {
                      tunnel: [w274 w281] -> w265
                      tunnel: w268 -> [w272 w282]
                      tunnel: w267 -> [w271 w280]
                      tunnel: w266 -> [w270 w279]
                      frame False {
                        w273 = TRUE ("Do this?")
                        n126 = global read "static dac defaults.vi" "Port 2"() -> (w277:i32)
                        n127 = Add(x=w271, y=w272) -> (x+y=w275:dbl)
                        n128 = global read "static dac defaults.vi" "Line 2"() -> (w278:i32)
                        n129 = call "ttl on.vi"("Line"=w278, "Port"=w277, "Do this?"=w273, "Input"=w270, "Absolute start time (ms)"=w271) -> ("Output"=w276:i32[][])
                        n130 = call "ttl off.vi"("Line"=w278, "Port"=w277, "Do this?"=w273, "Input"=w276, "Absolute start time (ms)"=w275) -> ("Output"=w274:i32[][])
                      }
                      frame True {
                        w283 = TRUE ("Do this?")
                        n131 = global read "static dac defaults.vi" "Port"() -> (w285:i32)
                        n132 = Add(x=w280, y=w282) -> (x+y=w287:dbl)
                        n133 = global read "static dac defaults.vi" "Line"() -> (w284:i32)
                        n134 = call "ttl on.vi"("Line"=w284, "Port"=w285, "Do this?"=w283, "Input"=w279, "Absolute start time (ms)"=w280) -> ("Output"=w286:i32[][])
                        n135 = call "ttl off.vi"("Line"=w284, "Port"=w285, "Do this?"=w283, "Input"=w286, "Absolute start time (ms)"=w287) -> ("Output"=w281:i32[][])
                      }
                    }
                  }
                  n136 = Insert Into Array(array=w259, new element=w258) -> (w254:dbl[])  [unwired: 1 in]
                  n137 = Insert Into Array(array=w260, new element=w246) -> (w256:dbl[])  [unwired: 1 in]
                  n138 = Array Size(array=w254) -> (size(s)=w253:i32)
                  n139 = Bundle By Name(cluster=w261, "Times"=w256, "Voltages"=w254, "Enable Ch"=TRUE, "Hinge Points"=w253) -> (w255:T10)
                }
              }
            }
          }
        }
      }
      "Output" <- w101
      "Static output" <- w103
      "GPIB Output" <- w96
    }
  }
